vi "Main.vi"() -> ()   [LabVIEW 2025]
uses:
  lib/Serial Data.ctl
  <vilib>/Utility/error.llb/Trim Whitespace One-Sided.vi
  <vilib>/Instr/_visa.llb/VISA Configure Serial Port (Instr).vi
panel:
  in  "Baud Rate":u32=9600
  in  "Serial Port":refnum<visa-resource-name>
  in  "stop program":bool
  in  "Send new sensor settings":bool
  in  "LDR's Detection Factor":dbl
  in  "Ultrasonic max distance":dbl
  out "Map":picture
  in  "Write Serial Data String":string
  in  "Read Serial Data":T1
  in  "Write Serial Data":T1
  in  "Read Serial Data String":string
  in  "Regions":enum32{"Region 1", "Region 2", "Region 3"}(tab)
  in  "Automatic Control 1":bool
  in  "Traffic Flow Control 1":dbl
  out "Traffic Flow Graph 1":dbl[](graph) caption="Traffic Flow"
  in  "Close Traffic Light 2":bool
  in  "Open Traffic Light 2":bool
  out "Green 2":bool
  out "Yellow 2":bool
  out "Red 2":bool
  in  "Close Traffic Light 1":bool
  in  "Open Traffic Light 1":bool
  out "Green 1":bool
  out "Yellow 1":bool
  out "Red 1":bool
  in  "Traffic Flow Control 2":dbl
  in  "Automatic Control 2":bool
  out "Traffic Flow Graph 2":dbl[](graph) caption="Traffic Flow"
  in  "Close Traffic Light 3":bool
  in  "Open Traffic Light 3":bool
  out "Green 3":bool
  out "Yellow 3":bool
  out "Red 3":bool
  in  "Traffic Flow Control 3":dbl
  in  "Automatic Control 3":bool
  out "Traffic Flow Graph 3":dbl[](graph) caption="Traffic Flow"
  in  "Close Traffic Light 4":bool
  in  "Open Traffic Light 4":bool
  out "Green 4":bool
  out "Yellow 4":bool
  out "Red 4":bool
  # "Comunicação Serial"
  # "Taxa de transmissão"
  # "Porta Serial"
  # "Sensores"
  # "Fator de detecção do LDR(%)"
  # "Distância máxima do ultrassônico(cm)"
  # "Fluxo de trânsito (carros/min)"
  # "Ativar controle automático"
  # "S2"
  # "S1"
  # "Fluxo de trânsito (carros/min)"
  # "Ativar controle automático"
  # "S3"
  # "Fluxo de trânsito (carros/min)"
  # "Ativar controle automático"
  # "S4"
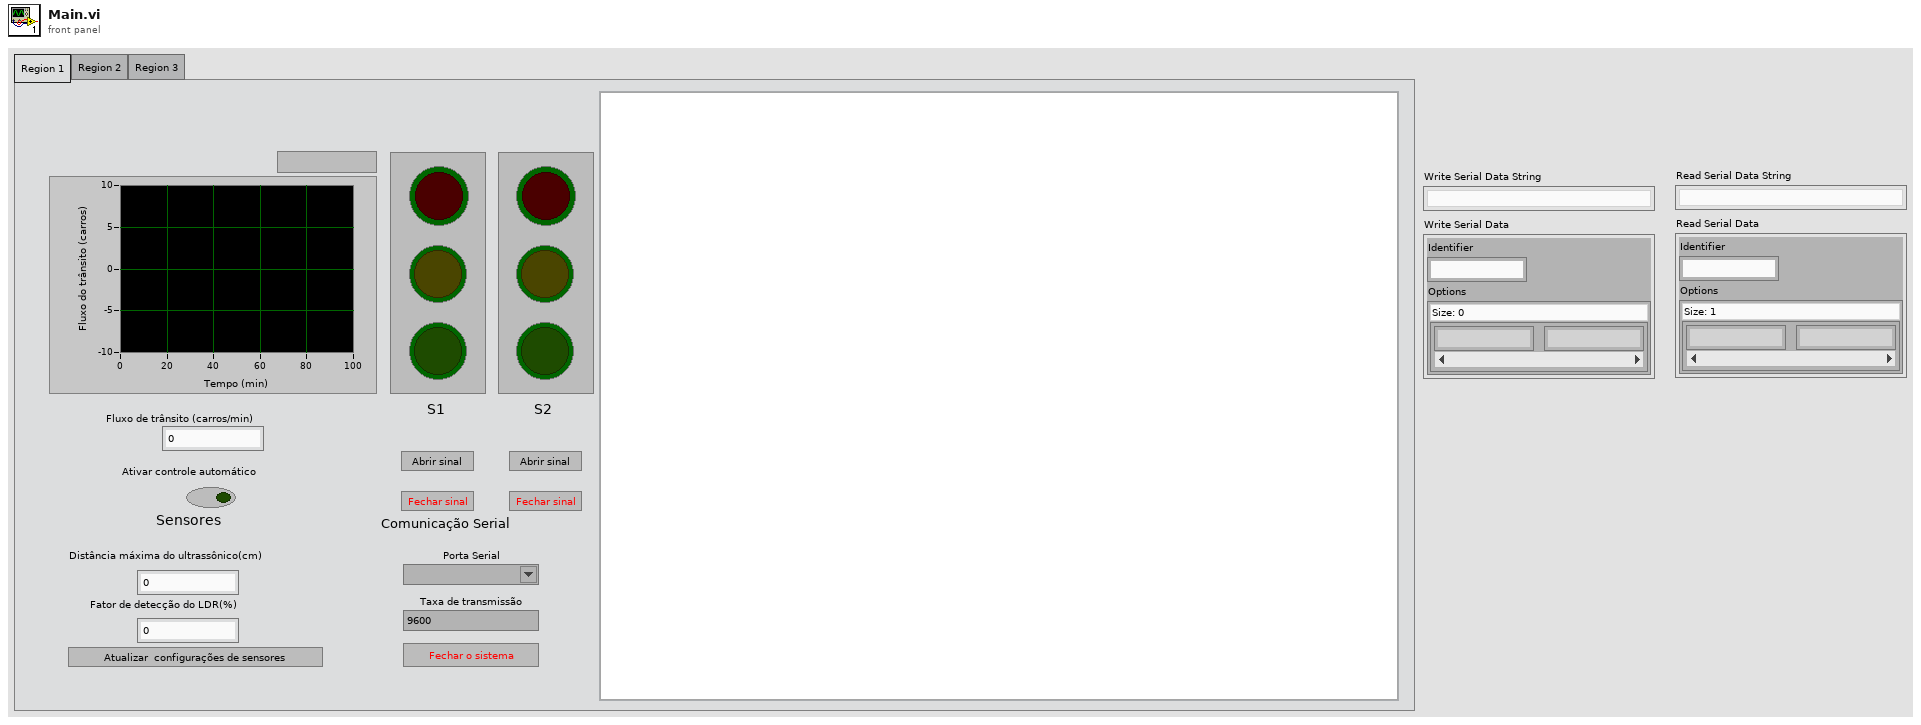
[diagram p1: front panel]
types:
  T1 = typedef "Serial Data.ctl" = cluster{"Identifier":string, "Options":map{string, string}}
  T2 = typedef "imagedata.ctl" = cluster{"image type":i32, "image depth":i32, "image":u8[], "mask":u8[], "colors":u32[], "Rectangle":cluster{"left":i16, "top":i16, "right":i16, "bottom":i16}}
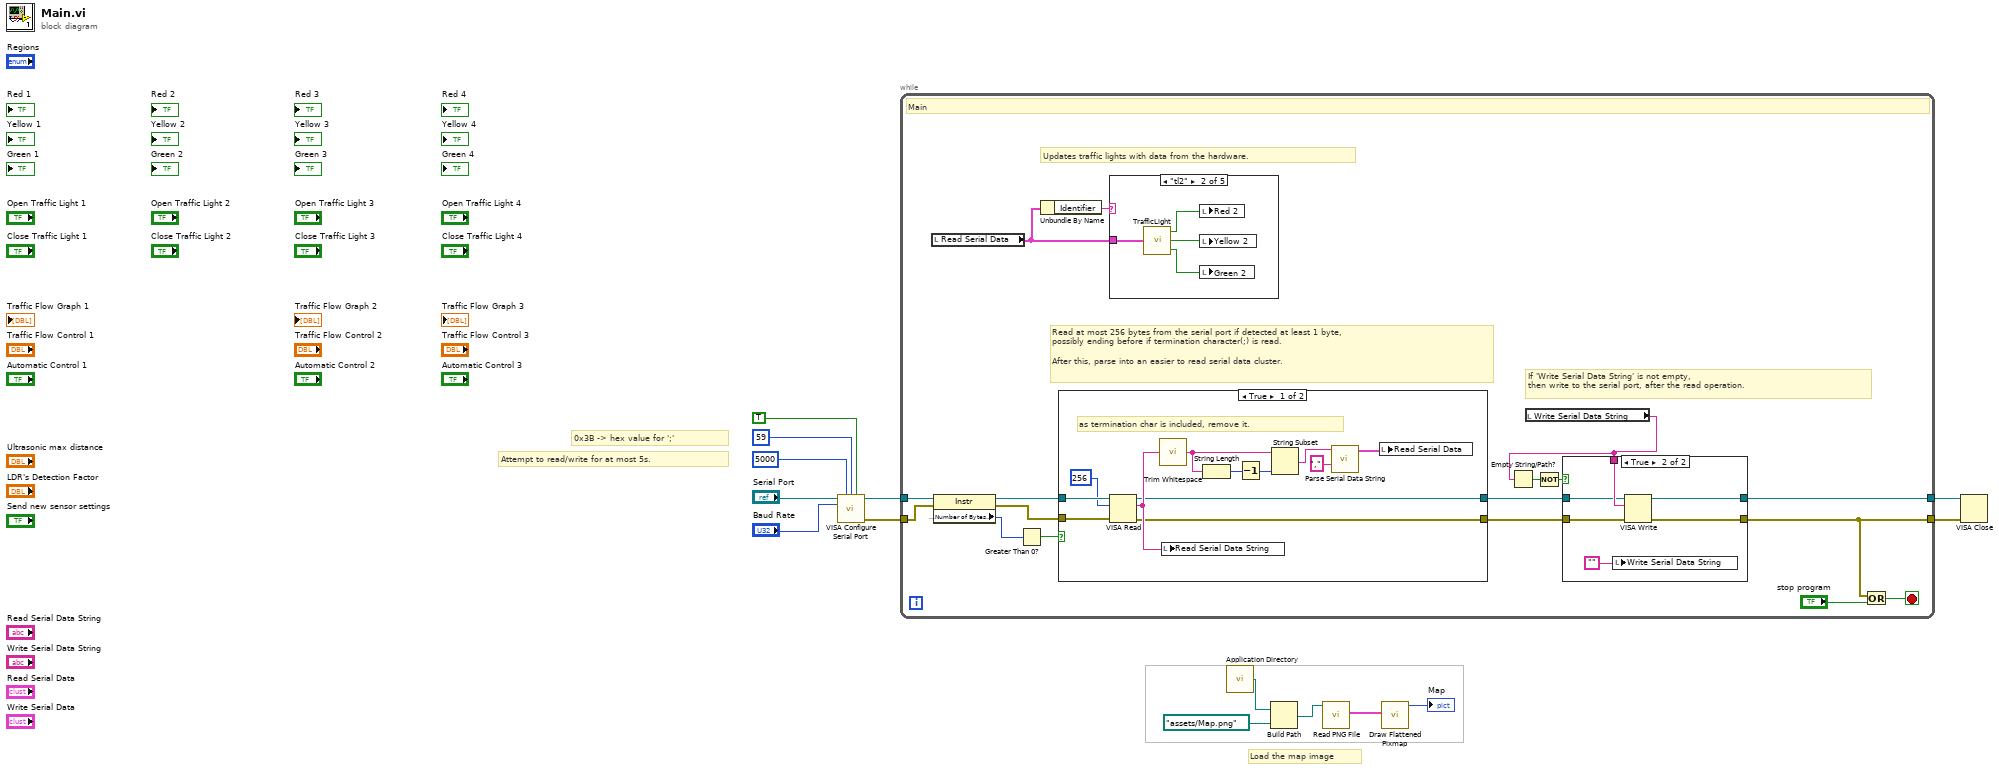
[diagram p0: block diagram]
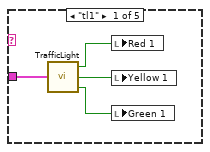
[diagram p2: hidden frame]
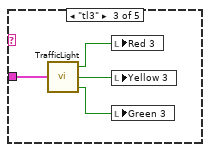
[diagram p3: hidden frame]
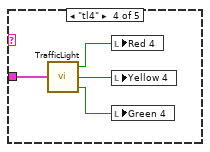
[diagram p4: hidden frame]
diagram:
  # "Attempt to read/write for at most 5s."
  # "Load the map image"
  # "0x3B -> hex value for ';'"
  n1 = call-poly "VISA Configure Serial Port"("VISA resource name"="Serial Port", "timeout (10sec)"=u32 5000, "termination char\n(0xA = '\\n' = LF)"=u8 59 ("termination char\n(0xA = '\\n' = LF)"), "Enable Termination\nChar (T)"=TRUE ("Enable Termination\nChar (T)"), "baud rate (9600)"="Baud Rate") -> ("VISA resource name out"=w10:refnum<visa-resource-name>, "error out"=w9:errorcluster)  [unwired: 9 in]
  n2 = while {
    tunnel: w10 -> [w29]
    tunnel: w9 -> [w28]
    tunnel: [w17] -> w8
    tunnel: [w19] -> w7
    stop <- w31 stop-if-true
    # "Updates traffic lights with data from the hardware."
    # "Read at most 256 bytes from the serial port if detected at least 1 byte,\npossibly ending before if termination character(;) is read.\n\nAfter this, parse into an easier to read serial data cluster."
    # "If 'Write Serial Data String' is not empty,\nthen write to the serial port, after the read operation."
    # "Main"
    n3 = local read "Read Serial Data"() -> (w15:T1)
    n4 = property class="Instr"(reference=w29, error in=w28) -> (reference out=w27:refnum<visa-resource-name>, error out=w26:errorcluster, "Serial Settings:Number of Bytes at Serial Port"=w24:u32)
    n5 = Greater Than 0?(x=w24) -> (x > 0?=w25:bool)
    n6 = Unbundle By Name(w15) -> ("Identifier"=w16:string)
    n7 = case shown="True" w25 {
      tunnel: w27 -> [w63 w69]
      tunnel: w26 -> [w62 w68]
      tunnel: [w61 w68] -> w20
      tunnel: [w60 w69] -> w21
      frame True {
        # "as termination char is included, remove it."
        n8 = VISA Read(VISA resource name=w63, byte count=u32 256, error in (no error)=w62) -> (VISA resource name out=w60:refnum<visa-resource-name>, read buffer=w64:string, error out=w61:errorcluster)  [unwired: 1 out]
        n9 = call <vilib>:"Trim Whitespace.vi"("string"=w64) -> ("trimmed string"=w66:string)  [unwired: 1 in]
        n10 = local write "Read Serial Data String"(w64) -> ()
        n11 = String Length(string=w66) -> (length=w65:i32)
        n12 = Decrement(x=w65) -> (x-1=w67:i32)
        n13 = String Subset(string=w66, length (rest)=w67) -> (substring=w57:string)  [unwired: 1 in]
        n14 = call "Parse Serial Data String.vi"("delimiter"=",", "serial data string"=w57) -> ("parsed serial data"=w56:T1)  [unwired: 4 in]
        n15 = local write "Read Serial Data"(w56) -> ()
      }
      frame False {
      }
    }
    n16 = case shown="\"tl2\"" w16 {
      tunnel: w15 -> [w32 w36 w40 w44 _]
      frame "tl1" {
        n17 = call "TrafficLight.vi"("Serial Data"=w32) -> ("Green"=w33:bool, "Yellow"=w34:bool, "Red"=w35:bool)  [unwired: 2 in]
        n18 = local write "Red 1"(w35) -> ()
        n19 = local write "Yellow 1"(w34) -> ()
        n20 = local write "Green 1"(w33) -> ()
      }
      frame "tl2" {
        n21 = call "TrafficLight.vi"("Serial Data"=w36) -> ("Green"=w37:bool, "Yellow"=w38:bool, "Red"=w39:bool)  [unwired: 2 in]
        n22 = local write "Red 2"(w39) -> ()
        n23 = local write "Yellow 2"(w38) -> ()
        n24 = local write "Green 2"(w37) -> ()
      }
      frame "tl3" {
        n25 = call "TrafficLight.vi"("Serial Data"=w40) -> ("Green"=w41:bool, "Yellow"=w42:bool, "Red"=w43:bool)  [unwired: 2 in]
        n26 = local write "Red 3"(w43) -> ()
        n27 = local write "Yellow 3"(w42) -> ()
        n28 = local write "Green 3"(w41) -> ()
      }
      frame "tl4" {
        n29 = call "TrafficLight.vi"("Serial Data"=w44) -> ("Green"=w45:bool, "Yellow"=w46:bool, "Red"=w47:bool)  [unwired: 2 in]
        n30 = local write "Red 4"(w47) -> ()
        n31 = local write "Yellow 4"(w46) -> ()
        n32 = local write "Green 4"(w45) -> ()
      }
      frame Default {
      }
    }
    n33 = local read "Write Serial Data String"() -> (w18:string)
    n34 = Empty String/Path?(string/path=w18) -> (empty?=w23:bool)
    n35 = Not(x=w23) -> (.not. x?=w22:bool)
    n36 = case shown="True" w22 {
      tunnel: w18 -> [_ w55]
      tunnel: w21 -> [w49 w54]
      tunnel: w20 -> [w48 w53]
      tunnel: [w49 w52] -> w19
      tunnel: [w48 w51] -> w17
      frame False {
      }
      frame True {
        n37 = local write "Write Serial Data String"("") -> ()
        n38 = VISA Write(VISA resource name=w54, write buffer=w55, error in (no error)=w53) -> (VISA resource name out=w52:refnum<visa-resource-name>, error out=w51:errorcluster)  [unwired: 1 out]
      }
    }
    n39 = Or(x=w17, y="stop program") -> (x .or. y?=w31:bool)
  }
  n40 = call <vilib>:"Application Directory.vi"() -> ("Application Directory"=w4:path)
  n41 = Build Path(base path=w4, name or relative path=path "assets/Map.png" ("Path")) -> (appended path=w2:path)
  n42 = call <vilib>:"Read PNG File.vi"("path to PNG file"=w2) -> ("image data"=w6:T2)  [unwired: 8 in, 2 out]
  n43 = call <vilib>:"Draw Flattened Pixmap.vi"("image data"=w6) -> ("new picture"=→"Map":picture)  [unwired: 8 in]
  n44 = VISA Close(VISA resource name=w7, error in (no error)=w8) -> ()  [unwired: 1 out]
